vi "Burst-Enumerate Valid Params.vi"(8 "error in (no error)":errorcluster, 11 "Burst":T1(xcontrol)) -> (0 "error out":errorcluster, 2 "Parameter Names":string[](array[string]))   [LabVIEW 2015]
uses:
  Controls/Burst XCtl/Burst Control.xctl
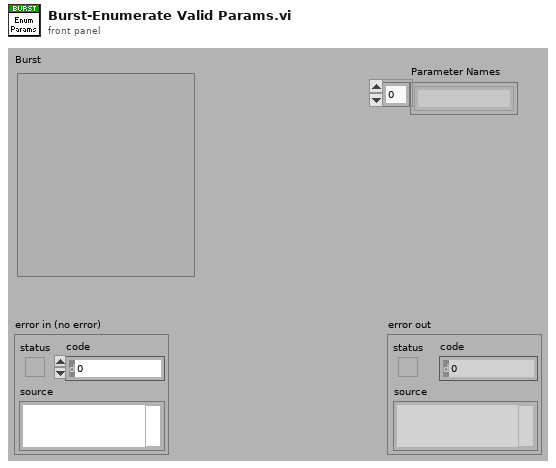
[diagram p1: front panel]
types:
  T1 = cluster{"Active":bool, "Delay (ms)":dbl, "Duration (ms)":dbl, "Ramp (ms)":dbl, "Rate (Hz)":dbl, "Trepeat (ms)":dbl, "Repeat":bool}
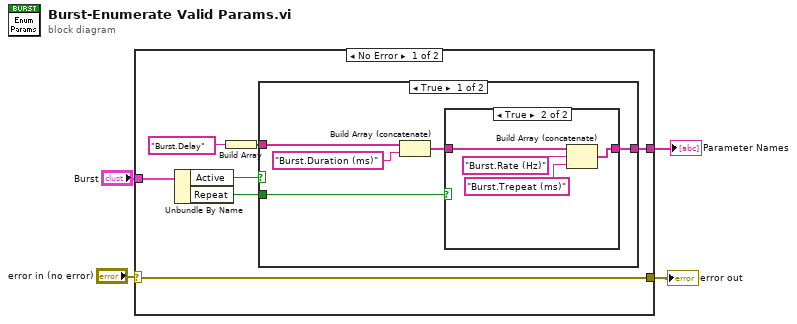
[diagram p0: block diagram]
diagram:
  n1 = case shown="No Error" "error in (no error)" {
    selector: "error in (no error)" -> [w9 w23]
    tunnel: "Burst" -> [w10 _]
    tunnel: [w9 w23] -> w2
    tunnel: [w5 _] -> w1
    frame No Error {
      n2 = Unbundle By Name(w10) -> ("Active"=w11:bool, "Repeat"=w8:bool)
      n3 = Build Array("Burst.Delay" ("String")) -> (w6:string[])
      n4 = case shown="True" w11 {
        tunnel: w8 -> [w14 _]
        tunnel: w6 -> [w15 w22]
        tunnel: [w12 w22] -> w5
        frame True {
          n5 = Build Array (concatenate)(w15, "Burst.Duration (ms)" ("String")) -> (w13:string[])
          n6 = case shown="True" w14 {
            tunnel: w13 -> [w17 w21]
            tunnel: [w17 w20] -> w12
            frame False {
            }
            frame True {
              n7 = Build Array (concatenate)(w21, "Burst.Rate (Hz)" ("String"), "Burst.Trepeat (ms)" ("String")) -> (w20:string[])
            }
          }
        }
        frame False {
        }
      }
    }
    frame Error {
    }
  }
  "error out" <- w2
  "Parameter Names" <- w1
